vi "setDefaultAmount.vi"(8 "error in (no error)":errorcluster, 10 "Default Amount":dbl, 11 "Category in":refnum<class "Category.lvclass">) -> (0 "error out":errorcluster, 3 "Category out":refnum<class "Category.lvclass">)   [LabVIEW 2018, in "Category.lvclass"]
uses:
  Category.lvclass
  Category.lvclass/Category.ctl
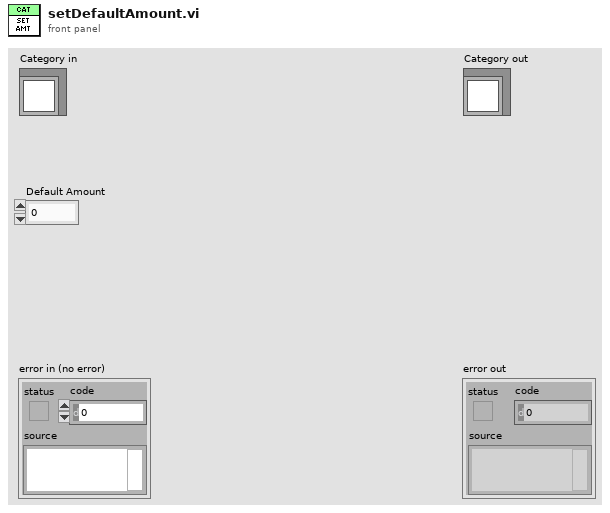
[diagram p1: front panel]
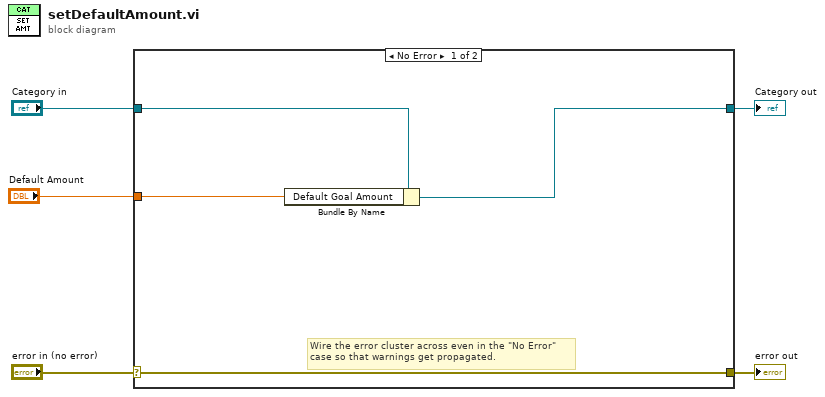
[diagram p0: block diagram]
diagram:
  n1 = case shown="No Error" "error in (no error)" {
    selector: "error in (no error)" -> [w9 w11]
    tunnel: [w9 w11] -> w4
    tunnel: [w7 w10] -> w2
    tunnel: "Category in" -> [w8 w10]
    tunnel: "Default Amount" -> [w6 _]
    frame No Error {
      # "Wire the error cluster across even in the \"No Error\"\ncase so that warnings get propagated."
      n2 = Bundle By Name(cluster=w8, "Default Goal Amount"=w6) -> (w7:refnum<class "Category.lvclass">)
    }
    frame Error {
    }
  }
  "error out" <- w4
  "Category out" <- w2
